vi "Mod_OFDM_Examine_Configure_OFDM_Symbol.vi"(0 "Configuration in":variant=variant("Data Source Pool "=variant(cluster{"mode (PN)":enum16{"PN", "pattern", "user"}, "PN sequence order (9)":i32, "base bit pattern (00001111)":enum16{"0", "1", "01", "0011", "00001111"}, "User base bit pattern":i8[]}[] [{"mode (PN)"=enum."PN", "PN sequence order (9)"=9, "base bit pattern (00001111)"=enum."00001111", "User base bit pattern"=[]}, {"mode (PN)"=enum."PN", "PN sequence order (9)"=9, "base bit pattern (00001111)"=enum."00001111", "User base bit pattern"=[]}, {"mode (PN)"=enum."PN", "PN sequence order (9)"=9, "base bit pattern (00001111)"=enum."00001111", "User base bit pattern"=[]}, {"mode (PN)"=enum."PN", "PN sequence order (9)"=9, "base bit pattern (00001111)"=enum."00001111", "User base bit pattern"=[]}, {"mode (PN)"=enum."PN", "PN sequence order (9)"=9, "base bit pattern (00001111)"=enum."00001111", "User base bit pattern"=[]}, {"mode (PN)"=enum."PN", "PN sequence order (9)"=9, "base bit pattern (00001111)"=enum."00001111", "User base bit pattern"=[]}]), "Modulator Source Pool "=variant(cluster{"M-QAM":enum16{"4", "16", "64", "256", "1024"}, "M-PSK":enum16{"2", "4", "8", "16", "32", "64", "128", "256"}, "Type of Modulation":enum16{"PSK", "QAM"}, "PSK":cluster{"differential PSK":enum16{"disable", "enable"}, "PSK type":u16}}[] [{"M-QAM"=enum."4", "M-PSK"=enum."4", "Type of Modulation"=enum."PSK", "PSK"={"differential PSK"=enum."disable", "PSK type"=0}}, {"M-QAM"=enum."4", "M-PSK"=enum."4", "Type of Modulation"=enum."PSK", "PSK"={"differential PSK"=enum."disable", "PSK type"=0}}, {"M-QAM"=enum."4", "M-PSK"=enum."4", "Type of Modulation"=enum."PSK", "PSK"={"differential PSK"=enum."disable", "PSK type"=0}}, {"M-QAM"=enum."4", "M-PSK"=enum."4", "Type of Modulation"=enum."PSK", "PSK"={"differential PSK"=enum."disable", "PSK type"=0}}, {"M-QAM"=enum."4", "M-PSK"=enum."4", "Type of Modulation"=enum."PSK", "PSK"={"differential PSK"=enum."disable", "PSK type"=0}}, {"M-QAM"=enum."4", "M-PSK"=enum."2", "Type of Modulation"=enum."PSK", "PSK"={"differential PSK"=enum."disable", "PSK type"=0}}]), "OFDM SYMBOL POOL"=variant(string[] []), "Sub Carrier Selection"=variant(cluster{"Sub Carrier":bool, "Data Source":u16, "Modulator":u16}[] [{"Sub Carrier"=TRUE, "Data Source"=0, "Modulator"=0}, {"Sub Carrier"=TRUE, "Data Source"=0, "Modulator"=0}, {"Sub Carrier"=TRUE, "Data Source"=0, "Modulator"=0}, {"Sub Carrier"=TRUE, "Data Source"=0, "Modulator"=0}, {"Sub Carrier"=TRUE, "Data Source"=0, "Modulator"=0}, {"Sub Carrier"=TRUE, "Data Source"=0, "Modulator"=0}, {"Sub Carrier"=TRUE, "Data Source"=0, "Modulator"=0}, {"Sub Carrier"=TRUE, "Data Source"=0, "Modulator"=0}, {"Sub Carrier"=TRUE, "Data Source"=0, "Modulator"=0}, {"Sub Carrier"=TRUE, "Data Source"=0, "Modulator"=0}, {"Sub Carrier"=TRUE, "Data Source"=0, "Modulator"=0}, {"Sub Carrier"=TRUE, "Data Source"=0, "Modulator"=0}, {"Sub Carrier"=TRUE, "Data Source"=0, "Modulator"=0}, {"Sub Carrier"=TRUE, "Data Source"=0, "Modulator"=0}, {"Sub Carrier"=TRUE, "Data Source"=0, "Modulator"=0}, {"Sub Carrier"=TRUE, "Data Source"=0, "Modulator"=0}, {"Sub Carrier"=TRUE, "Data Source"=0, "Modulator"=0}, {"Sub Carrier"=TRUE, "Data Source"=0, "Modulator"=0}, {"Sub Carrier"=TRUE, "Data Source"=0, "Modulator"=0}, {"Sub Carrier"=TRUE, "Data Source"=0, "Modulator"=0}, {"Sub Carrier"=TRUE, "Data Source"=0, "Modulator"=0}, {"Sub Carrier"=TRUE, "Data Source"=0, "Modulator"=0}, {"Sub Carrier"=TRUE, "Data Source"=0, "Modulator"=0}, {"Sub Carrier"=TRUE, "Data Source"=0, "Modulator"=0}, {"Sub Carrier"=TRUE, "Data Source"=0, "Modulator"=0}, {"Sub Carrier"=TRUE, "Data Source"=0, "Modulator"=0}, {"Sub Carrier"=TRUE, "Data Source"=0, "Modulator"=0}, {"Sub Carrier"=TRUE, "Data Source"=0, "Modulator"=0}, {"Sub Carrier"=TRUE, "Data Source"=0, "Modulator"=0}, {"Sub Carrier"=TRUE, "Data Source"=0, "Modulator"=0}, {"Sub Carrier"=TRUE, "Data Source"=0, "Modulator"=0}, {"Sub Carrier"=TRUE, "Data Source"=0, "Modulator"=0}, {"Sub Carrier"=TRUE, "Data Source"=0, "Modulator"=0}, {"Sub Carrier"=TRUE, "Data Source"=0, "Modulator"=0}, {"Sub Carrier"=TRUE, "Data Source"=0, "Modulator"=0}, {"Sub Carrier"=TRUE, "Data Source"=0, "Modulator"=0}, {"Sub Carrier"=TRUE, "Data Source"=0, "Modulator"=0}, {"Sub Carrier"=TRUE, "Data Source"=0, "Modulator"=0}, {"Sub Carrier"=TRUE, "Data Source"=0, "Modulator"=0}, {"Sub Carrier"=TRUE, "Data Source"=0, "Modulator"=0}, {"Sub Carrier"=TRUE, "Data Source"=0, "Modulator"=0}, {"Sub Carrier"=TRUE, "Data Source"=0, "Modulator"=0}, {"Sub Carrier"=TRUE, "Data Source"=0, "Modulator"=0}, {"Sub Carrier"=TRUE, "Data Source"=0, "Modulator"=0}, {"Sub Carrier"=TRUE, "Data Source"=0, "Modulator"=0}, {"Sub Carrier"=TRUE, "Data Source"=0, "Modulator"=0}, {"Sub Carrier"=TRUE, "Data Source"=0, "Modulator"=0}, {"Sub Carrier"=TRUE, "Data Source"=0, "Modulator"=0}, {"Sub Carrier"=TRUE, "Data Source"=0, "Modulator"=0}, {"Sub Carrier"=TRUE, "Data Source"=0, "Modulator"=0}, {"Sub Carrier"=TRUE, "Data Source"=0, "Modulator"=0}, {"Sub Carrier"=TRUE, "Data Source"=0, "Modulator"=0}, {"Sub Carrier"=TRUE, "Data Source"=0, "Modulator"=0}, {"Sub Carrier"=TRUE, "Data Source"=0, "Modulator"=0}, {"Sub Carrier"=TRUE, "Data Source"=0, "Modulator"=0}, {"Sub Carrier"=TRUE, "Data Source"=0, "Modulator"=0}, {"Sub Carrier"=TRUE, "Data Source"=0, "Modulator"=0}, {"Sub Carrier"=TRUE, "Data Source"=0, "Modulator"=0}, {"Sub Carrier"=TRUE, "Data Source"=0, "Modulator"=0}, {"Sub Carrier"=TRUE, "Data Source"=0, "Modulator"=0}, {"Sub Carrier"=TRUE, "Data Source"=0, "Modulator"=0}, {"Sub Carrier"=TRUE, "Data Source"=0, "Modulator"=0}, {"Sub Carrier"=TRUE, "Data Source"=0, "Modulator"=0}, {"Sub Carrier"=TRUE, "Data Source"=0, "Modulator"=0}, {"Sub Carrier"=TRUE, "Data Source"=0, "Modulator"=0}, {"Sub Carrier"=TRUE, "Data Source"=0, "Modulator"=0}, {"Sub Carrier"=TRUE, "Data Source"=0, "Modulator"=0}, {"Sub Carrier"=TRUE, "Data Source"=0, "Modulator"=0}, {"Sub Carrier"=TRUE, "Data Source"=0, "Modulator"=0}, {"Sub Carrier"=TRUE, "Data Source"=0, "Modulator"=0}, {"Sub Carrier"=TRUE, "Data Source"=0, "Modulator"=0}, {"Sub Carrier"=TRUE, "Data Source"=0, "Modulator"=0}, {"Sub Carrier"=TRUE, "Data Source"=0, "Modulator"=0}, {"Sub Carrier"=TRUE, "Data Source"=0, "Modulator"=0}, {"Sub Carrier"=TRUE, "Data Source"=0, "Modulator"=0}, {"Sub Carrier"=TRUE, "Data Source"=0, "Modulator"=0}, {"Sub Carrier"=TRUE, "Data Source"=0, "Modulator"=0}, {"Sub Carrier"=TRUE, "Data Source"=0, "Modulator"=0}, {"Sub Carrier"=TRUE, "Data Source"=0, "Modulator"=0}, {"Sub Carrier"=TRUE, "Data Source"=0, "Modulator"=0}, {"Sub Carrier"=TRUE, "Data Source"=0, "Modulator"=0}, {"Sub Carrier"=TRUE, "Data Source"=0, "Modulator"=0}, {"Sub Carrier"=TRUE, "Data Source"=0, "Modulator"=0}, {"Sub Carrier"=TRUE, "Data Source"=0, "Modulator"=0}, {"Sub Carrier"=TRUE, "Data Source"=0, "Modulator"=0}, {"Sub Carrier"=TRUE, "Data Source"=0, "Modulator"=0}, {"Sub Carrier"=TRUE, "Data Source"=0, "Modulator"=0}, {"Sub Carrier"=TRUE, "Data Source"=0, "Modulator"=0}, {"Sub Carrier"=TRUE, "Data Source"=0, "Modulator"=0}, {"Sub Carrier"=TRUE, "Data Source"=0, "Modulator"=0}, {"Sub Carrier"=TRUE, "Data Source"=0, "Modulator"=0}, {"Sub Carrier"=TRUE, "Data Source"=0, "Modulator"=0}, {"Sub Carrier"=TRUE, "Data Source"=0, "Modulator"=0}, {"Sub Carrier"=TRUE, "Data Source"=0, "Modulator"=0}, {"Sub Carrier"=TRUE, "Data Source"=0, "Modulator"=0}, {"Sub Carrier"=TRUE, "Data Source"=0, "Modulator"=0}, {"Sub Carrier"=TRUE, "Data Source"=0, "Modulator"=0}, {"Sub Carrier"=TRUE, "Data Source"=0, "Modulator"=0}, {"Sub Carrier"=TRUE, "Data Source"=0, "Modulator"=0}, {"Sub Carrier"=TRUE, "Data Source"=0, "Modulator"=0}, {"Sub Carrier"=TRUE, "Data Source"=0, "Modulator"=0}, {"Sub Carrier"=TRUE, "Data Source"=0, "Modulator"=0}, {"Sub Carrier"=TRUE, "Data Source"=0, "Modulator"=0}, {"Sub Carrier"=TRUE, "Data Source"=0, "Modulator"=0}, {"Sub Carrier"=TRUE, "Data Source"=0, "Modulator"=0}, {"Sub Carrier"=TRUE, "Data Source"=0, "Modulator"=0}, {"Sub Carrier"=TRUE, "Data Source"=0, "Modulator"=0}, {"Sub Carrier"=TRUE, "Data Source"=0, "Modulator"=0}, {"Sub Carrier"=TRUE, "Data Source"=0, "Modulator"=0}, {"Sub Carrier"=TRUE, "Data Source"=0, "Modulator"=0}, {"Sub Carrier"=TRUE, "Data Source"=0, "Modulator"=0}, {"Sub Carrier"=TRUE, "Data Source"=0, "Modulator"=0}, {"Sub Carrier"=TRUE, "Data Source"=0, "Modulator"=0}, {"Sub Carrier"=TRUE, "Data Source"=0, "Modulator"=0}, {"Sub Carrier"=TRUE, "Data Source"=0, "Modulator"=0}, {"Sub Carrier"=TRUE, "Data Source"=0, "Modulator"=0}, {"Sub Carrier"=TRUE, "Data Source"=0, "Modulator"=0}, {"Sub Carrier"=TRUE, "Data Source"=0, "Modulator"=0}, {"Sub Carrier"=TRUE, "Data Source"=0, "Modulator"=0}, {"Sub Carrier"=TRUE, "Data Source"=0, "Modulator"=0}, {"Sub Carrier"=TRUE, "Data Source"=0, "Modulator"=0}, {"Sub Carrier"=TRUE, "Data Source"=0, "Modulator"=0}, {"Sub Carrier"=TRUE, "Data Source"=0, "Modulator"=0}, {"Sub Carrier"=TRUE, "Data Source"=0, "Modulator"=0}, {"Sub Carrier"=TRUE, "Data Source"=0, "Modulator"=0}, {"Sub Carrier"=TRUE, "Data Source"=0, "Modulator"=0}, {"Sub Carrier"=TRUE, "Data Source"=0, "Modulator"=0}, {"Sub Carrier"=TRUE, "Data Source"=0, "Modulator"=0}]), "Symbol Table"=variant(string[][] [])), 11 "error in":errorcluster) -> (4 "Configuration out":variant=variant("Data Source Pool "=variant(cluster{"mode (PN)":enum16{"PN", "pattern", "user"}, "PN sequence order (9)":i32, "base bit pattern (00001111)":enum16{"0", "1", "01", "0011", "00001111"}, "User base bit pattern":i8[]}[] [{"mode (PN)"=enum."PN", "PN sequence order (9)"=9, "base bit pattern (00001111)"=enum."00001111", "User base bit pattern"=[]}, {"mode (PN)"=enum."PN", "PN sequence order (9)"=9, "base bit pattern (00001111)"=enum."00001111", "User base bit pattern"=[]}, {"mode (PN)"=enum."PN", "PN sequence order (9)"=9, "base bit pattern (00001111)"=enum."00001111", "User base bit pattern"=[]}, {"mode (PN)"=enum."PN", "PN sequence order (9)"=9, "base bit pattern (00001111)"=enum."00001111", "User base bit pattern"=[]}, {"mode (PN)"=enum."PN", "PN sequence order (9)"=9, "base bit pattern (00001111)"=enum."00001111", "User base bit pattern"=[]}, {"mode (PN)"=enum."PN", "PN sequence order (9)"=9, "base bit pattern (00001111)"=enum."00001111", "User base bit pattern"=[]}]), "Modulator Source Pool "=variant(cluster{"M-QAM":enum16{"4", "16", "64", "256", "1024"}, "M-PSK":enum16{"2", "4", "8", "16", "32", "64", "128", "256"}, "Type of Modulation":enum16{"PSK", "QAM"}, "PSK":cluster{"differential PSK":enum16{"disable", "enable"}, "PSK type":u16}}[] [{"M-QAM"=enum."4", "M-PSK"=enum."4", "Type of Modulation"=enum."PSK", "PSK"={"differential PSK"=enum."disable", "PSK type"=0}}, {"M-QAM"=enum."4", "M-PSK"=enum."4", "Type of Modulation"=enum."PSK", "PSK"={"differential PSK"=enum."disable", "PSK type"=0}}, {"M-QAM"=enum."4", "M-PSK"=enum."4", "Type of Modulation"=enum."PSK", "PSK"={"differential PSK"=enum."disable", "PSK type"=0}}, {"M-QAM"=enum."4", "M-PSK"=enum."4", "Type of Modulation"=enum."PSK", "PSK"={"differential PSK"=enum."disable", "PSK type"=0}}, {"M-QAM"=enum."4", "M-PSK"=enum."4", "Type of Modulation"=enum."PSK", "PSK"={"differential PSK"=enum."disable", "PSK type"=0}}, {"M-QAM"=enum."4", "M-PSK"=enum."2", "Type of Modulation"=enum."PSK", "PSK"={"differential PSK"=enum."disable", "PSK type"=0}}]), "OFDM SYMBOL POOL"=variant(string[] []), "Sub Carrier Selection"=variant(cluster{"Sub Carrier":bool, "Data Source":u16, "Modulator":u16}[] [{"Sub Carrier"=TRUE, "Data Source"=0, "Modulator"=0}, {"Sub Carrier"=TRUE, "Data Source"=0, "Modulator"=0}, {"Sub Carrier"=TRUE, "Data Source"=0, "Modulator"=0}, {"Sub Carrier"=TRUE, "Data Source"=0, "Modulator"=0}, {"Sub Carrier"=TRUE, "Data Source"=0, "Modulator"=0}, {"Sub Carrier"=TRUE, "Data Source"=0, "Modulator"=0}, {"Sub Carrier"=TRUE, "Data Source"=0, "Modulator"=0}, {"Sub Carrier"=TRUE, "Data Source"=0, "Modulator"=0}, {"Sub Carrier"=TRUE, "Data Source"=0, "Modulator"=0}, {"Sub Carrier"=TRUE, "Data Source"=0, "Modulator"=0}, {"Sub Carrier"=TRUE, "Data Source"=0, "Modulator"=0}, {"Sub Carrier"=TRUE, "Data Source"=0, "Modulator"=0}, {"Sub Carrier"=TRUE, "Data Source"=0, "Modulator"=0}, {"Sub Carrier"=TRUE, "Data Source"=0, "Modulator"=0}, {"Sub Carrier"=TRUE, "Data Source"=0, "Modulator"=0}, {"Sub Carrier"=TRUE, "Data Source"=0, "Modulator"=0}, {"Sub Carrier"=TRUE, "Data Source"=0, "Modulator"=0}, {"Sub Carrier"=TRUE, "Data Source"=0, "Modulator"=0}, {"Sub Carrier"=TRUE, "Data Source"=0, "Modulator"=0}, {"Sub Carrier"=TRUE, "Data Source"=0, "Modulator"=0}, {"Sub Carrier"=TRUE, "Data Source"=0, "Modulator"=0}, {"Sub Carrier"=TRUE, "Data Source"=0, "Modulator"=0}, {"Sub Carrier"=TRUE, "Data Source"=0, "Modulator"=0}, {"Sub Carrier"=TRUE, "Data Source"=0, "Modulator"=0}, {"Sub Carrier"=TRUE, "Data Source"=0, "Modulator"=0}, {"Sub Carrier"=TRUE, "Data Source"=0, "Modulator"=0}, {"Sub Carrier"=TRUE, "Data Source"=0, "Modulator"=0}, {"Sub Carrier"=TRUE, "Data Source"=0, "Modulator"=0}, {"Sub Carrier"=TRUE, "Data Source"=0, "Modulator"=0}, {"Sub Carrier"=TRUE, "Data Source"=0, "Modulator"=0}, {"Sub Carrier"=TRUE, "Data Source"=0, "Modulator"=0}, {"Sub Carrier"=TRUE, "Data Source"=0, "Modulator"=0}, {"Sub Carrier"=TRUE, "Data Source"=0, "Modulator"=0}, {"Sub Carrier"=TRUE, "Data Source"=0, "Modulator"=0}, {"Sub Carrier"=TRUE, "Data Source"=0, "Modulator"=0}, {"Sub Carrier"=TRUE, "Data Source"=0, "Modulator"=0}, {"Sub Carrier"=TRUE, "Data Source"=0, "Modulator"=0}, {"Sub Carrier"=TRUE, "Data Source"=0, "Modulator"=0}, {"Sub Carrier"=TRUE, "Data Source"=0, "Modulator"=0}, {"Sub Carrier"=TRUE, "Data Source"=0, "Modulator"=0}, {"Sub Carrier"=TRUE, "Data Source"=0, "Modulator"=0}, {"Sub Carrier"=TRUE, "Data Source"=0, "Modulator"=0}, {"Sub Carrier"=TRUE, "Data Source"=0, "Modulator"=0}, {"Sub Carrier"=TRUE, "Data Source"=0, "Modulator"=0}, {"Sub Carrier"=TRUE, "Data Source"=0, "Modulator"=0}, {"Sub Carrier"=TRUE, "Data Source"=0, "Modulator"=0}, {"Sub Carrier"=TRUE, "Data Source"=0, "Modulator"=0}, {"Sub Carrier"=TRUE, "Data Source"=0, "Modulator"=0}, {"Sub Carrier"=TRUE, "Data Source"=0, "Modulator"=0}, {"Sub Carrier"=TRUE, "Data Source"=0, "Modulator"=0}, {"Sub Carrier"=TRUE, "Data Source"=0, "Modulator"=0}, {"Sub Carrier"=TRUE, "Data Source"=0, "Modulator"=0}, {"Sub Carrier"=TRUE, "Data Source"=0, "Modulator"=0}, {"Sub Carrier"=TRUE, "Data Source"=0, "Modulator"=0}, {"Sub Carrier"=TRUE, "Data Source"=0, "Modulator"=0}, {"Sub Carrier"=TRUE, "Data Source"=0, "Modulator"=0}, {"Sub Carrier"=TRUE, "Data Source"=0, "Modulator"=0}, {"Sub Carrier"=TRUE, "Data Source"=0, "Modulator"=0}, {"Sub Carrier"=TRUE, "Data Source"=0, "Modulator"=0}, {"Sub Carrier"=TRUE, "Data Source"=0, "Modulator"=0}, {"Sub Carrier"=TRUE, "Data Source"=0, "Modulator"=0}, {"Sub Carrier"=TRUE, "Data Source"=0, "Modulator"=0}, {"Sub Carrier"=TRUE, "Data Source"=0, "Modulator"=0}, {"Sub Carrier"=TRUE, "Data Source"=0, "Modulator"=0}, {"Sub Carrier"=TRUE, "Data Source"=0, "Modulator"=0}, {"Sub Carrier"=TRUE, "Data Source"=0, "Modulator"=0}, {"Sub Carrier"=TRUE, "Data Source"=0, "Modulator"=0}, {"Sub Carrier"=TRUE, "Data Source"=0, "Modulator"=0}, {"Sub Carrier"=TRUE, "Data Source"=0, "Modulator"=0}, {"Sub Carrier"=TRUE, "Data Source"=0, "Modulator"=0}, {"Sub Carrier"=TRUE, "Data Source"=0, "Modulator"=0}, {"Sub Carrier"=TRUE, "Data Source"=0, "Modulator"=0}, {"Sub Carrier"=TRUE, "Data Source"=0, "Modulator"=0}, {"Sub Carrier"=TRUE, "Data Source"=0, "Modulator"=0}, {"Sub Carrier"=TRUE, "Data Source"=0, "Modulator"=0}, {"Sub Carrier"=TRUE, "Data Source"=0, "Modulator"=0}, {"Sub Carrier"=TRUE, "Data Source"=0, "Modulator"=0}, {"Sub Carrier"=TRUE, "Data Source"=0, "Modulator"=0}, {"Sub Carrier"=TRUE, "Data Source"=0, "Modulator"=0}, {"Sub Carrier"=TRUE, "Data Source"=0, "Modulator"=0}, {"Sub Carrier"=TRUE, "Data Source"=0, "Modulator"=0}, {"Sub Carrier"=TRUE, "Data Source"=0, "Modulator"=0}, {"Sub Carrier"=TRUE, "Data Source"=0, "Modulator"=0}, {"Sub Carrier"=TRUE, "Data Source"=0, "Modulator"=0}, {"Sub Carrier"=TRUE, "Data Source"=0, "Modulator"=0}, {"Sub Carrier"=TRUE, "Data Source"=0, "Modulator"=0}, {"Sub Carrier"=TRUE, "Data Source"=0, "Modulator"=0}, {"Sub Carrier"=TRUE, "Data Source"=0, "Modulator"=0}, {"Sub Carrier"=TRUE, "Data Source"=0, "Modulator"=0}, {"Sub Carrier"=TRUE, "Data Source"=0, "Modulator"=0}, {"Sub Carrier"=TRUE, "Data Source"=0, "Modulator"=0}, {"Sub Carrier"=TRUE, "Data Source"=0, "Modulator"=0}, {"Sub Carrier"=TRUE, "Data Source"=0, "Modulator"=0}, {"Sub Carrier"=TRUE, "Data Source"=0, "Modulator"=0}, {"Sub Carrier"=TRUE, "Data Source"=0, "Modulator"=0}, {"Sub Carrier"=TRUE, "Data Source"=0, "Modulator"=0}, {"Sub Carrier"=TRUE, "Data Source"=0, "Modulator"=0}, {"Sub Carrier"=TRUE, "Data Source"=0, "Modulator"=0}, {"Sub Carrier"=TRUE, "Data Source"=0, "Modulator"=0}, {"Sub Carrier"=TRUE, "Data Source"=0, "Modulator"=0}, {"Sub Carrier"=TRUE, "Data Source"=0, "Modulator"=0}, {"Sub Carrier"=TRUE, "Data Source"=0, "Modulator"=0}, {"Sub Carrier"=TRUE, "Data Source"=0, "Modulator"=0}, {"Sub Carrier"=TRUE, "Data Source"=0, "Modulator"=0}, {"Sub Carrier"=TRUE, "Data Source"=0, "Modulator"=0}, {"Sub Carrier"=TRUE, "Data Source"=0, "Modulator"=0}, {"Sub Carrier"=TRUE, "Data Source"=0, "Modulator"=0}, {"Sub Carrier"=TRUE, "Data Source"=0, "Modulator"=0}, {"Sub Carrier"=TRUE, "Data Source"=0, "Modulator"=0}, {"Sub Carrier"=TRUE, "Data Source"=0, "Modulator"=0}, {"Sub Carrier"=TRUE, "Data Source"=0, "Modulator"=0}, {"Sub Carrier"=TRUE, "Data Source"=0, "Modulator"=0}, {"Sub Carrier"=TRUE, "Data Source"=0, "Modulator"=0}, {"Sub Carrier"=TRUE, "Data Source"=0, "Modulator"=0}, {"Sub Carrier"=TRUE, "Data Source"=0, "Modulator"=0}, {"Sub Carrier"=TRUE, "Data Source"=0, "Modulator"=0}, {"Sub Carrier"=TRUE, "Data Source"=0, "Modulator"=0}, {"Sub Carrier"=TRUE, "Data Source"=0, "Modulator"=0}, {"Sub Carrier"=TRUE, "Data Source"=0, "Modulator"=0}, {"Sub Carrier"=TRUE, "Data Source"=0, "Modulator"=0}, {"Sub Carrier"=TRUE, "Data Source"=0, "Modulator"=0}, {"Sub Carrier"=TRUE, "Data Source"=0, "Modulator"=0}, {"Sub Carrier"=TRUE, "Data Source"=0, "Modulator"=0}, {"Sub Carrier"=TRUE, "Data Source"=0, "Modulator"=0}, {"Sub Carrier"=TRUE, "Data Source"=0, "Modulator"=0}, {"Sub Carrier"=TRUE, "Data Source"=0, "Modulator"=0}, {"Sub Carrier"=TRUE, "Data Source"=0, "Modulator"=0}, {"Sub Carrier"=TRUE, "Data Source"=0, "Modulator"=0}]), "Symbol Table"=variant(string[][] [["0", " ON", "0", "1"], ["1", " ON", "0", "1"], ["2", " ON", "0", "1"], ["3", " ON", "0", "1"], ["4", " ON", "0", "1"], ["5", " ON", "0", "1"], ["6", " ON", "0", "1"], ["7", " ON", "0", "1"], ["8", " ON", "0", "1"], ["9", " ON", "0", "1"], ["10", " ON", "0", "1"], ["11", " ON", "0", "1"], ["12", " ON", "0", "1"], ["13", " ON", "0", "1"], ["14", " ON", "0", "1"], ["15", " ON", "0", "1"], ["16", " ON", "0", "1"], ["17", " ON", "0", "1"], ["18", " ON", "0", "1"], ["19", " ON", "0", "1"], ["20", " ON", "0", "1"], ["21", " ON", "0", "1"], ["22", " ON", "0", "1"], ["23", " ON", "0", "1"], ["24", " ON", "0", "1"], ["25", " ON", "0", "1"], ["26", " ON", "0", "1"], ["27", " ON", "0", "1"], ["28", " ON", "0", "1"], ["29", " ON", "0", "1"], ["30", " ON", "0", "1"], ["31", " ON", "0", "1"], ["32", " ON", "0", "1"], ["33", " ON", "0", "1"], ["34", " ON", "0", "1"], ["35", " ON", "0", "1"], ["36", " ON", "0", "1"], ["37", " ON", "0", "1"], ["38", " ON", "0", "1"], ["39", " ON", "0", "1"], ["40", " ON", "0", "1"], ["41", " ON", "0", "1"], ["42", " ON", "0", "1"], ["43", " ON", "0", "1"], ["44", " ON", "0", "1"], ["45", " ON", "0", "1"], ["46", " ON", "0", "1"], ["47", " ON", "0", "1"], ["48", " ON", "0", "1"], ["49", " ON", "0", "1"], ["50", " ON", "0", "1"], ["51", " ON", "0", "1"], ["52", " ON", "0", "1"], ["53", " ON", "0", "1"], ["54", " ON", "0", "1"], ["55", " ON", "0", "1"], ["56", " ON", "0", "1"], ["57", " ON", "0", "1"], ["58", " ON", "0", "1"], ["59", " ON", "0", "1"], ["60", " ON", "0", "1"], ["61", " ON", "0", "1"], ["62", " ON", "0", "1"], ["63", " ON", "0", "1"]])), 15 "error out":errorcluster)   [LabVIEW 2010]
doc: "The VI allows to examine/configure the OFDM symbol structure. The user can define prototypes of the OFDM symbols that are required to be generated and/or stored (in a file). These prototypes are kept in a pool which are used to build the OFDM Frame. \n\nThe VI shows the current OFDM symbol structure in a table format, where each sub carrier information is displayed. The user can assign a data source and modulator source to a subcarrier from the pool of data sources and pool of modulator sources available."
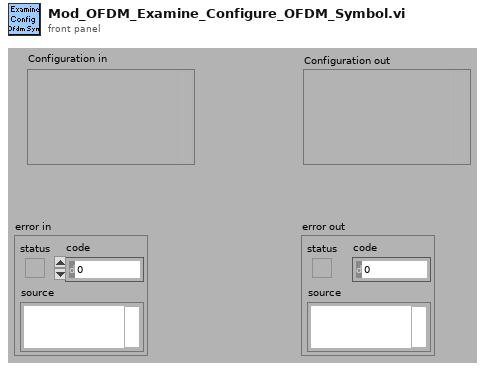
[diagram p1: front panel]
types:
  T1 = cluster{"# of Sub Carrier":i32, "Length Of Cylic Prefix":i32}
  T2 = typedef "Pool of Data Source Control.ctl" = cluster{"mode (PN)":enum16{"PN", "pattern", "user"}, "PN sequence order (9)":i32, "Invert Output Bits":enum16{"No", "Yes"}, "Register Initial State ":u32, "User base bit pattern":i8[], "base bit pattern (00001111)":enum16{"0", "1", "01", "0011", "00001111"}, "Reset to Initial State":enum16{"Every OFDM Frame", "Every OFDM Symbol", "Every Sub Carrier"}}[]
  T3 = typedef "Pool of Modulator Control.ctl" = cluster{"M-QAM":enum16{"4", "16", "64", "256"}, "M-PSK":enum16{"2", "4", "8", "16", "32", "64", "128", "256"}, "Type of Modulation":enum16{"PSK", "QAM"}, " PSK":cluster{"differential PSK":enum16{"disable", "enable"}, "PSK type":enum16{"normal", "shifted", "offset"}}}[]
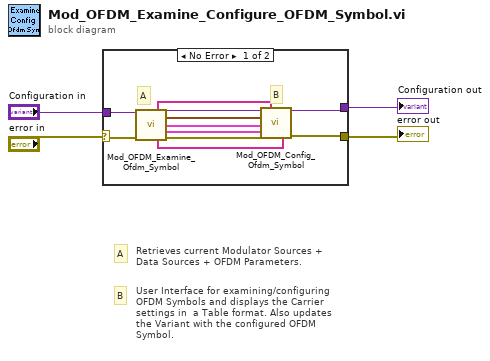
[diagram p0: block diagram]
diagram:
  # "User Interface for examining/configuring OFDM Symbols and displays the Carrier settings in  a Table format. Also updates  the Variant with the configured OFDM Symbol."
  # "Retrieves current Modulator Sources + Data Sources + OFDM Parameters."
  # "A"
  # "B"
  n1 = case shown="No Error" "error in" {
    selector: "error in" -> [w9 w16]
    tunnel: "Configuration in" -> [w15 _]
    tunnel: [w11 w16] -> w3
    tunnel: [w10 _] -> w2
    frame No Error {
      # "B"
      # "A"
      n2 = call "Mod_OFDM_Examine_Ofdm_Symbol.vi"("Configuration in"=w15, "error in"=w9) -> ("Data Source Names"=w6:string[], "Configuration out"=w13:variant, "OFDM Parameters"=w5:T1, "DATA Source Pool"=w8:T2, "Modulator Pool"=w7:T3, "Mod Names"=w14:string[], "error out"=w12:errorcluster)  [unwired: 7 in]
      n3 = call "Mod_OFDM_Config_Ofdm_Symbol.vi"("Configuration in"=w13, "Data Source Name"=w6, "OFDM PARAMETERS"=w5, "DATA Source Pool"=w8, "Modulator Pool"=w7, "error in"=w12, "Modulator Source Name"=w14) -> ("Configuration out"=w10:variant, "error out"=w11:errorcluster)  [unwired: 7 in]
    }
    frame Error {
    }
  }
  "error out" <- w3
  "Configuration out" <- w2
